vi "Load Settings.vi"(6 "Elso?":i32, 7 "Config":T1={"Hardware"={"VISA resource name"="COM3"}, "Logging"={"tdms file out"=refnum, "base path"=path ""}, "Set Temp"={"Numeric"=0.0}}, 8 "error constant":errorcluster) -> (0 "error constant 2":errorcluster, 5 "Config 2":T1)   [LabVIEW 2022 SP3]
uses:
  <vilib>/Utility/xml.llb/Read From XML File(string).vi
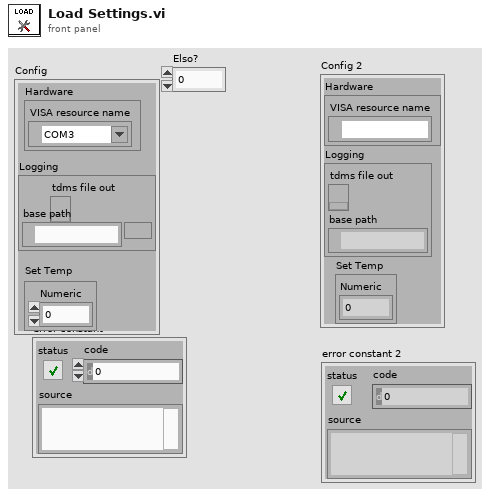
[diagram p1: front panel]
types:
  T1 = cluster{"Hardware":cluster{"VISA resource name":refnum<visa-resource-name>}, "Logging":cluster{"tdms file out":refnum<k34>, "base path":path}, "Set Temp":cluster{"Numeric":dbl}}
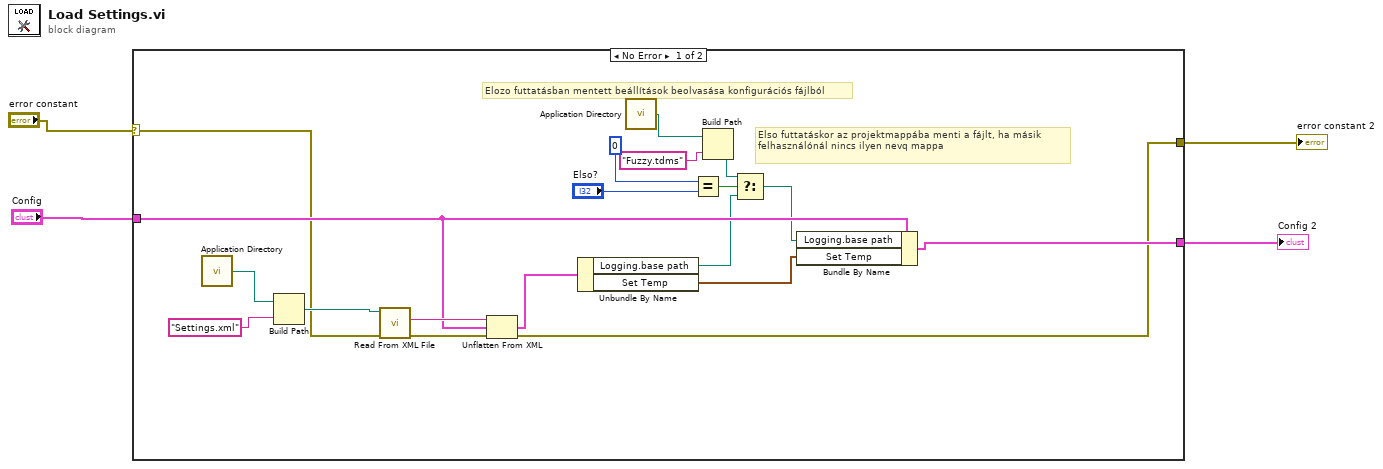
[diagram p0: block diagram]
diagram:
  n1 = case shown="No Error" "error constant" {
    selector: "error constant" -> [w15 w25]
    tunnel: "Config" -> [w18 w24]
    tunnel: [w16 w24] -> w2
    tunnel: [w13 w25] -> w1
    frame No Error {
      # "Elso futtatáskor az projektmappába menti a fájlt, ha másik felhasználónál nincs ilyen nevq mappa"
      # "Elozo futtatásban mentett beállítások beolvasása konfigurációs fájlból"
      n2 = call <vilib>:"Application Directory.vi"() -> ("Application Directory"=w23:path)
      n3 = Build Path(base path=w23, name or relative path="Settings.xml") -> (appended path=w21:path)
      n4 = call-poly <vilib>:"Read From XML File.vi"("error in (no error)"=w15, "XML File Path"=w21) -> ("error out"=w14:errorcluster, "XML Elements"=w20:string)  [unwired: 7 in, 1 out]
      n5 = Unflatten From XML(xml string=w20, type=w18, error in (no error)=w14) -> (value=w19:T1, error out=w13:errorcluster)
      n6 = Unbundle By Name(w19) -> ("Logging.base path"=w5:path, "Set Temp"=w17:cluster{"Numeric":dbl})
      n7 = call <vilib>:"Application Directory.vi"() -> ("Application Directory"=w8:path)
      n8 = Equal?(x=0, y="Elso?") -> (x = y?=w12:bool)
      n9 = Build Path(base path=w8, name or relative path="Fuzzy.tdms") -> (appended path=w9:path)
      n10 = Select(t=w9, s=w12, f=w5) -> (s? t:f=w6:path)
      n11 = Bundle By Name(cluster=w18, "Logging.base path"=w6, "Set Temp"=w17) -> (w16:T1)
    }
    frame Error {
    }
  }
  "error constant 2" <- w1
  "Config 2" <- w2
